vi "Draw Joint_picture.vi"(6 "JointType":i32(ring) items=["SpineBase", "SpineMid", "Neck", "Head", "ShoulderLeft", "ElbowLeft", "WristLeft", "HandLeft", "ShoulderRight", "ElbowRight", "WristRight", "HandRight", "HipLeft", "KneeLeft", "AnkleLeft", "FootLeft", "HipRight", "KneeRight", "AnkleRight", "FootRight", "SpineShoulder", "HandTipLeft", "ThumbLeft", "HandTipRight", "ThumbRight"], 8 "error in":errorcluster, 11 "picture":picture) -> (0 "error out":errorcluster, 3 "picture out":picture)   [LabVIEW 2014]
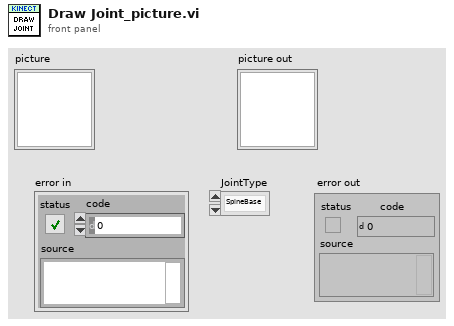
[diagram p1: front panel]
types:
  T1 = cluster{"Width":u16, "Style":enum32{"Solid", "Dash", "Dot", "DashDot", "DashDotDot"}}
  T2 = enum16{"Get Attribute", "Initialize", "Set Attribute"}
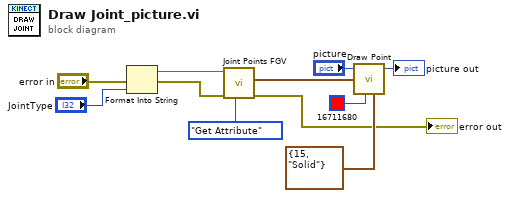
[diagram p0: block diagram]
diagram:
  n1 = Format Into String(error in="error in", "JointType") -> (resulting string=w9:string, error out=w8:errorcluster)  [unwired: 2 in]
  n2 = call "Joint Points FGV.vi"("Command"=T2."Get Attribute", "error in (no error)"=w8, "name"=w9) -> ("error out"=→"error out":errorcluster, "Joint Point"=w6:cluster{"X":sgl, "Y":sgl})  [unwired: 7 in]
  n3 = call <vilib>:"Draw Point.vi"("picture"="picture", "point(x,y)"=w6, "color(black)"=u32 16711680, "pen"=T1 {"Width"=15, "Style"=enum."Solid"}) -> ("new picture"=→"picture out":picture)  [unwired: 5 in]
